vi "P2 CALCOLATOR.vi"(4 "RPM":dbl, 5 "C[Nm]":dbl, 6 "Calcolo P2":T1(ring)=enum."coeff p2", 7 "Rend motore %":dbl, 8 "curva rendimento motore":dbl[][](array[numeric]), 9 "Coefficienti P2":enum32{"Radio Selection 1", "Radio Selection 2"}(radio), 10 "Coefficenti P2":T2, 11 "P1  kw":dbl) -> (3 "P2":dbl)   [LabVIEW 2019]
uses:
  <vilib>/Analysis/NI_AALPro.lvlib
  <vilib>/gmath/NI_Gmath.lvlib
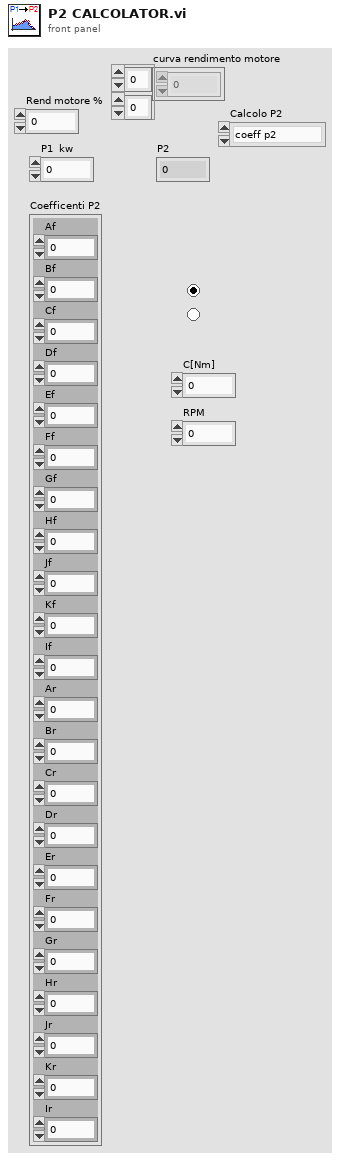
[diagram p1: front panel]
types:
  T1 = enum32{"Torsiometro", "coeff p2", "Rendimento", "Curva rend"}
  T2 = cluster{"Af":dbl, "Bf":dbl, "Cf":dbl, "Df":dbl, "Ef":dbl, "Ff":dbl, "Gf":dbl, "Hf":dbl, "Jf":dbl, "Kf":dbl, "If":dbl, "Ar":dbl, "Br":dbl, "Cr":dbl, "Dr":dbl, "Er":dbl, "Fr":dbl, "Gr":dbl, "Hr":dbl, "Jr":dbl, "Kr":dbl, "Ir":dbl}
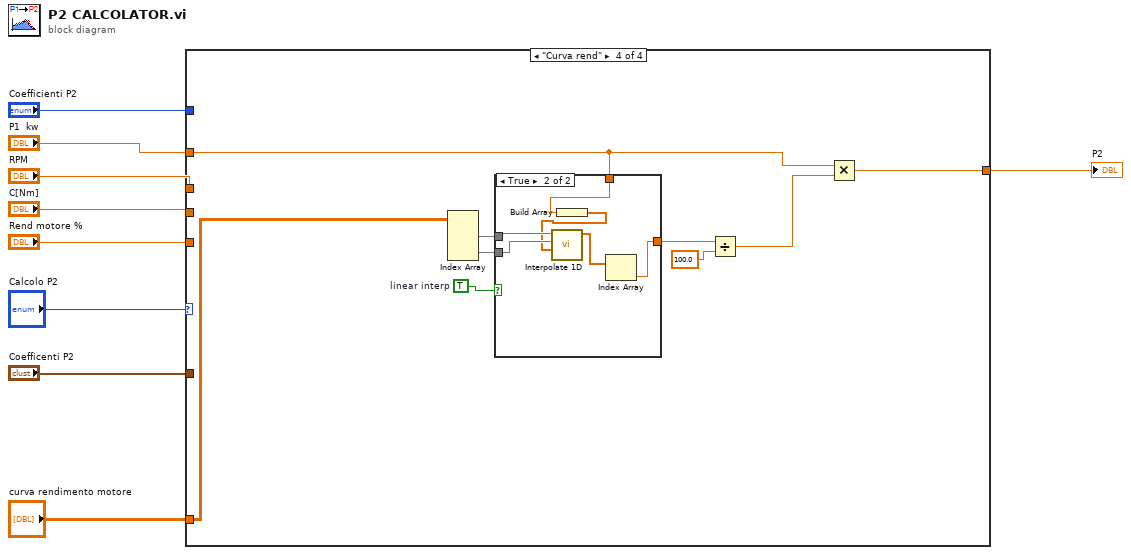
[diagram p0: block diagram]
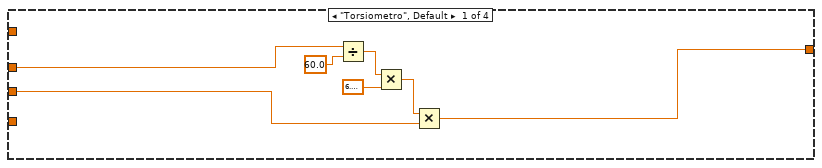
[diagram p2: hidden frame]
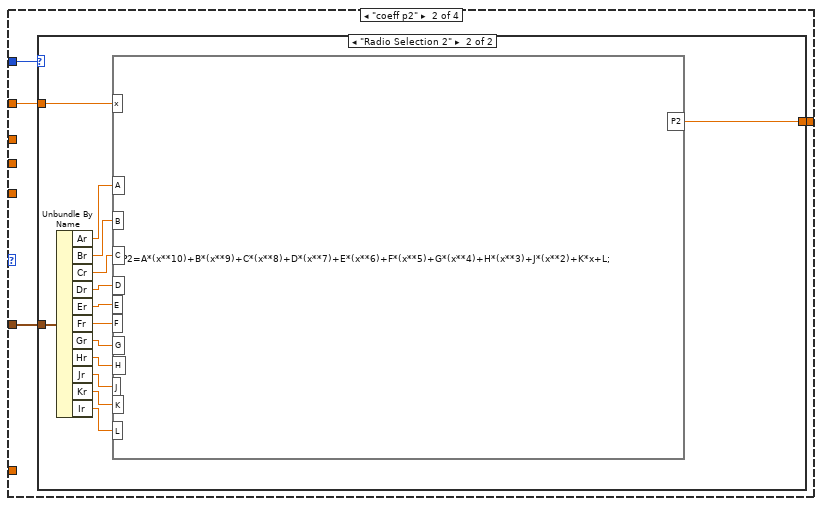
[diagram p3: hidden frame]
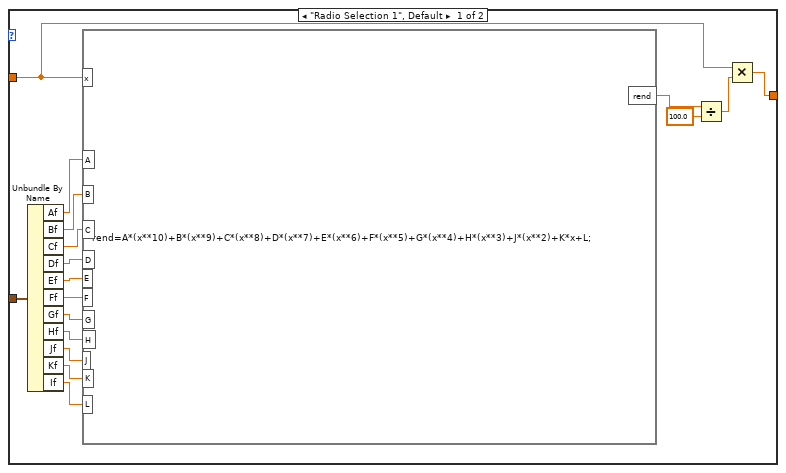
[diagram p4: hidden frame]
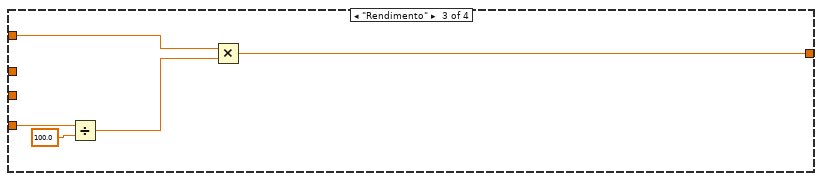
[diagram p5: hidden frame]
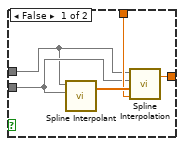
[diagram p6: hidden frame]
diagram:
  n1 = case shown="\"Curva rend\"" "Calcolo P2" {
    tunnel: "Coefficenti P2" -> [_ w20 _ _]
    tunnel: [w12 w19 w52 w60] -> w8
    tunnel: "P1  kw" -> [_ w18 w53 w62]
    tunnel: "Coefficienti P2" -> [_ w17 _ _]
    tunnel: "Rend motore %" -> [_ _ w56 _]
    tunnel: "curva rendimento motore" -> [_ _ _ w65]
    tunnel: "RPM" -> [w11 _ _ _]
    tunnel: "C[Nm]" -> [w10 _ _ _]
    frame "Torsiometro", Default {
      n2 = Divide(x=w11, y=60.0) -> (x/y=w15:dbl)
      n3 = Multiply(x=w15, y=6.283185307179586) -> (x*y=w13:dbl)
      n4 = Multiply(x=w13, y=w10) -> (x*y=w12:dbl)
    }
    frame "coeff p2" {
      n5 = case shown="\"Radio Selection 2\"" w17 {
        tunnel: w20 -> [w37 w51]
        tunnel: [w21 w39] -> w19
        tunnel: w18 -> [w22 w38]
        frame "Radio Selection 1", Default {
          n6 = Unbundle By Name(w37) -> ("Af"=w36:dbl, "Bf"=w35:dbl, "Cf"=w34:dbl, "Df"=w33:dbl, "Ef"=w32:dbl, "Ff"=w31:dbl, "Gf"=w30:dbl, "Hf"=w29:dbl, "Jf"=w28:dbl, "Kf"=w27:dbl, "If"=w26:dbl)
          n7 = formula code="rend=A*(x**10)+B*(x**9)+C*(x**8)+D*(x**7)+E*(x**6)+F*(x**5)+G*(x**4)+H*(x**3)+J*(x**2)+K*x+L;"("A"=w36, "B"=w35, "C"=w34, "D"=w33, "E"=w32, "F"=w31, "G"=w30, "H"=w29, "J"=w28, "K"=w27, "L"=w26, "x"=w22) -> ("rend"=w25:dbl)
          n8 = Divide(x=w25, y=100.0) -> (x/y=w23:dbl)
          n9 = Multiply(x=w22, y=w23) -> (x*y=w21:dbl)
        }
        frame "Radio Selection 2" {
          n10 = Unbundle By Name(w51) -> ("Ar"=w50:dbl, "Br"=w49:dbl, "Cr"=w48:dbl, "Dr"=w47:dbl, "Er"=w46:dbl, "Fr"=w45:dbl, "Gr"=w44:dbl, "Hr"=w43:dbl, "Jr"=w42:dbl, "Kr"=w41:dbl, "Ir"=w40:dbl)
          n11 = formula code="P2=A*(x**10)+B*(x**9)+C*(x**8)+D*(x**7)+E*(x**6)+F*(x**5)+G*(x**4)+H*(x**3)+J*(x**2)+K*x+L;"("A"=w50, "B"=w49, "C"=w48, "D"=w47, "E"=w46, "F"=w45, "G"=w44, "H"=w43, "J"=w42, "K"=w41, "L"=w40, "x"=w38) -> ("P2"=w39:dbl)
        }
      }
    }
    frame "Rendimento" {
      n12 = Divide(x=w56, y=100.0) -> (x/y=w54:dbl)
      n13 = Multiply(x=w53, y=w54) -> (x*y=w52:dbl)
    }
    frame "Curva rend" {
      w57 = TRUE  # linear interp
      n14 = Index Array(array=w65) -> (element #1=w58:dbl[], element #2=w59:dbl[])  [unwired: 4 in]
      n15 = case shown="True" w57 {
        tunnel: [w69 w71] -> w64
        tunnel: w62 -> [w68 w74]
        tunnel: w59 -> [w67 w75]
        tunnel: w58 -> [w66 w76]
        frame False {
          n16 = call <vilib>:"Spline Interpolant.vi"("X"=w67, "Y"=w66) -> ("Interpolant"=w70:dbl[])  [unwired: 2 in, 1 out]
          n17 = call <vilib>:"Spline Interpolation.vi"("x value"=w68, "Interpolant"=w70, "X"=w67, "Y"=w66) -> ("interpolation value"=w69:dbl)  [unwired: 1 out]
        }
        frame True {
          n18 = Build Array(w74) -> (w73:dbl[])
          n19 = call <vilib>:"Interpolate 1D.vi"("xi"=w73, "X"=w75, "Y"=w76) -> ("yi"=w72:dbl[])  [unwired: 6 in, 2 out]
          n20 = Index Array(array=w72) -> (element=w71:dbl)  [unwired: 1 in]
        }
      }
      n21 = Divide(x=w64, y=100.0) -> (x/y=w61:dbl)
      n22 = Multiply(x=w62, y=w61) -> (x*y=w60:dbl)
    }
  }
  "P2" <- w8
